vi "Update.vi"(9 "log line":string, 10 "file ref":refnum<file>, 11 "rollover trigger in":refnum<class "RolloverTrigger.lvclass">) -> (3 "rollover trigger out":refnum<class "RolloverTrigger.lvclass">)   [LabVIEW 2018, in "GLog.lvlib" / "RolloverTrigger.lvclass"]
doc: "Updates the internal state of the rollover trigger after the file is written to."
uses:
  RolloverTrigger.lvclass
panel:
  # "Connector Pane"
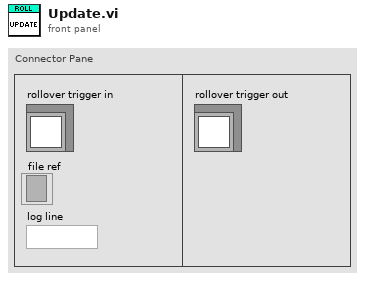
[diagram p1: front panel]
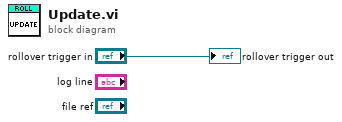
[diagram p0: block diagram]
diagram:
  "rollover trigger out" <- "rollover trigger in"
